vi "User32dllAPI.GetWindowPos.vi"(8 "error in (no error)":errorcluster, 11 "hWnd in":i32) -> (0 "error out":errorcluster, 2 "WinPos":T1, 3 "hWnd out":i32)   [LabVIEW 2019, in "Tools.lvlib"]
uses:
  Tools.lvlib
  user32.dll
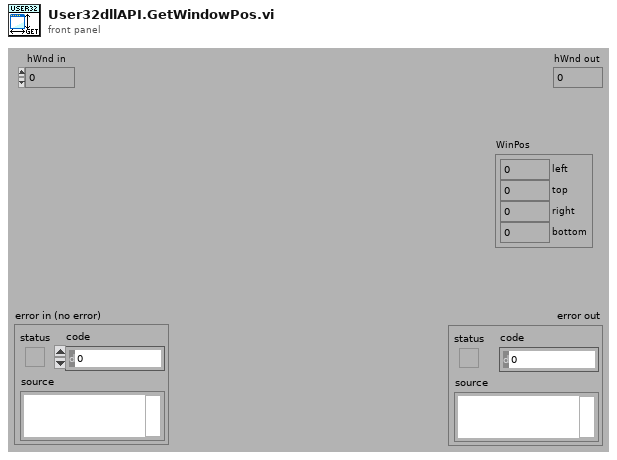
[diagram p1: front panel]
types:
  T1 = cluster{"left":i32, "top":i32, "right":i32, "bottom":i32}
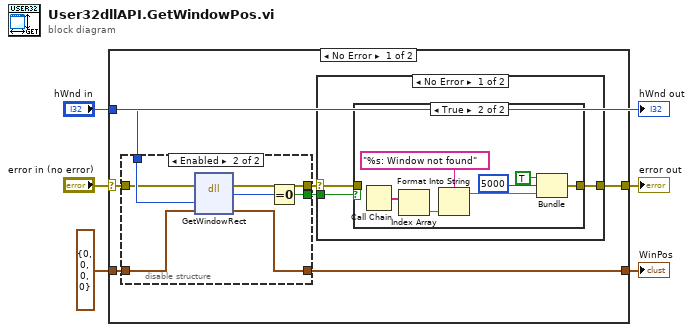
[diagram p0: block diagram]
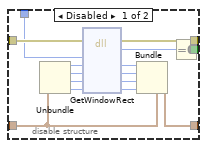
[diagram p2: hidden frame]
diagram:
  n1 = case shown="No Error" "error in (no error)" {
    selector: "error in (no error)" -> [w10 w48]
    tunnel: [w11 w48] -> w4
    tunnel: "hWnd in" -> [w7 _]
    tunnel: [w6 w47] -> w3
    tunnel: cluster{"X":i32, "Y":i32, "dX":i32, "dY":i32} {"X"=0, "Y"=0, "dX"=0, "dY"=0} ("WinPos") -> [w8 w47]
    frame No Error {
      n2 = disable-structure shown="Enabled" {
        disable-tunnel: [w27 w30] -> w12
        disable-tunnel: w10 -> [w26 w32]
        disable-tunnel: [w25 w31] -> w9
        disable-tunnel: w8 -> [w15 w34]
        disable-tunnel: w7 -> [w14 w33]
        disable-tunnel: [w13 w28] -> w6
        frame Disabled {
          n3 = Unbundle(w15) -> ("X"=w23:i32, "Y"=w22:i32, "dX"=w21:i32, "dY"=w20:i32)
          n4 = dll-call lib="user32.dll" fn="GetWindowRect"(error in=w26, "hWnd"=w14, "left"=w23, "top"=w22, "right"=w21, "bottom"=w20) -> (error out=w25:errorcluster, "bool"=w24:i32, "left"=w19:i32, "top"=w18:i32, "right"=w17:i32, "bottom"=w16:i32)  [unwired: 3 in, 1 out]
          n5 = Bundle(cluster=w15, "X"=w19, "Y"=w18, "dX"=w17, "dY"=w16) -> (w13:cluster{"X":i32, "Y":i32, "dX":i32, "dY":i32})
          n6 = Equal To 0?(x=w24) -> (x = 0?=w27:bool)
        }
        frame Enabled {
          n7 = dll-call lib="user32.dll" fn="GetWindowRect"(error in=w32, "hWnd"=w33, "left"=w34) -> (error out=w31:errorcluster, "bool"=w29:i32, "left"=w28:cluster{"X":i32, "Y":i32, "dX":i32, "dY":i32})  [unwired: 3 in, 1 out]
          n8 = Equal To 0?(x=w29) -> (x = 0?=w30:bool)
        }
      }
      n9 = case shown="No Error" w9 {
        selector: w9 -> [w35 w46]
        tunnel: w12 -> [w37 _]
        tunnel: [w36 w46] -> w11
        frame No Error {
          n10 = case shown="True" w37 {
            tunnel: [w38 w39] -> w36
            tunnel: w35 -> [w38 _]
            frame False {
            }
            frame True {
              n11 = Call Chain() -> (call chain=w45:string[])
              n12 = Index Array(array=w45) -> (element=w44:string)  [unwired: 1 in]
              n13 = Format Into String(format string="%s: Window not found", w44) -> (resulting string=w42:string)  [unwired: 2 in, 1 out]
              n14 = Bundle("status"=TRUE, "code"=5000, w42) -> (w39:cluster{"status":bool, "code":i32, string})  [unwired: 1 in]
            }
          }
        }
        frame Error {
        }
      }
    }
    frame Error {
    }
  }
  "error out" <- w4
  "WinPos" <- w3
  "hWnd out" <- "hWnd in"
